vi "N664_Init.vi"() -> (1 "Status":bool, 2 "Positions":dbl[](array[numeric]), 3 "VISA Refnum out":refnum<visa-resource-name>)   [LabVIEW 2014]
uses:
  <vilib>/Instr/_visa.llb/VISA Configure Serial Port (Instr).vi
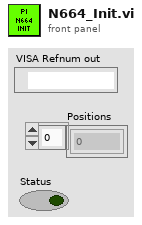
[diagram p1: front panel]
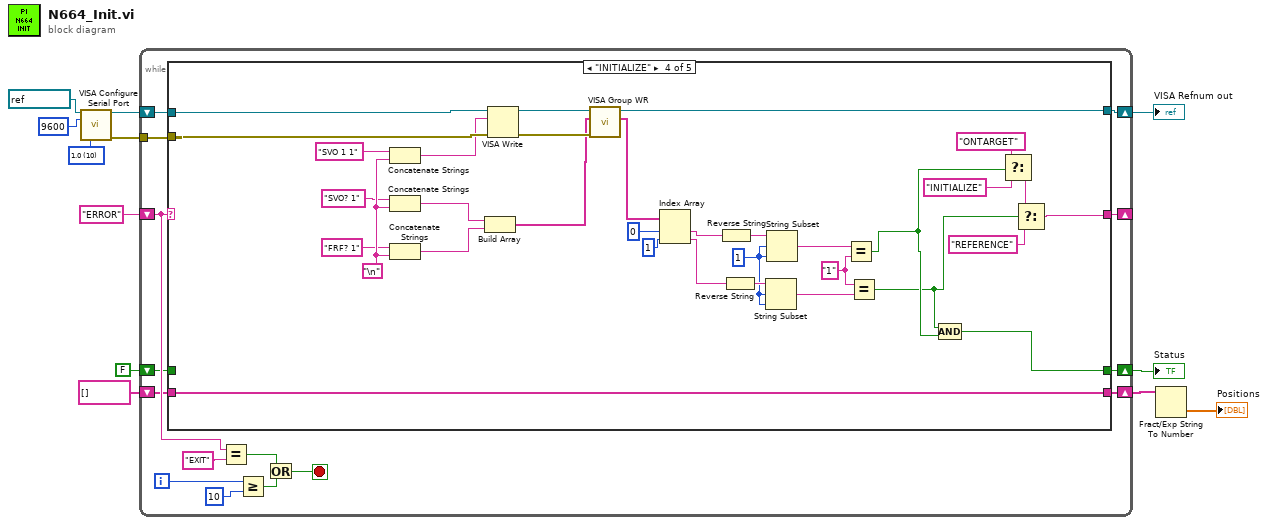
[diagram p0: block diagram]
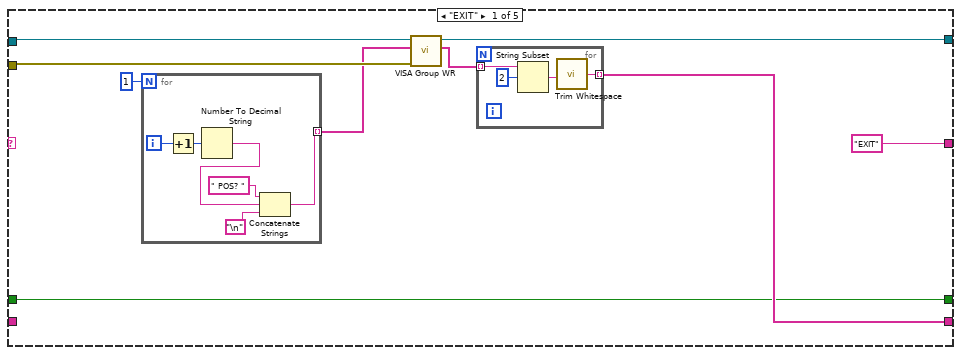
[diagram p2: hidden frame]
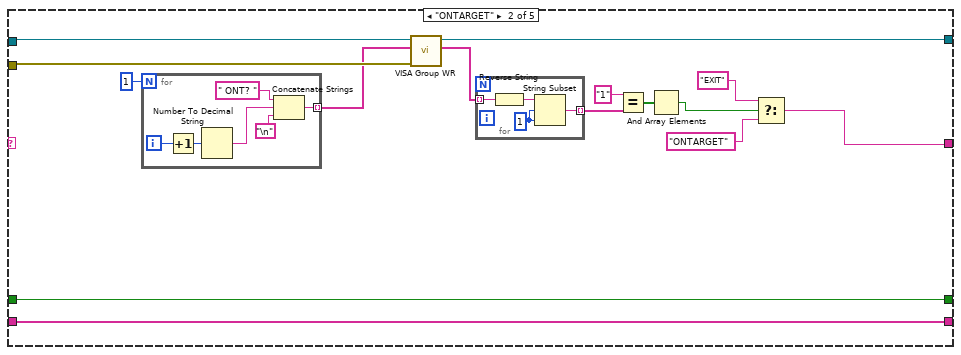
[diagram p3: hidden frame]
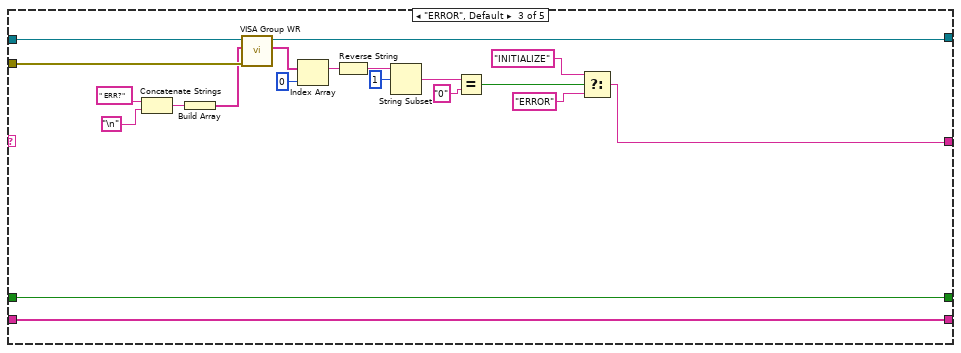
[diagram p4: hidden frame]
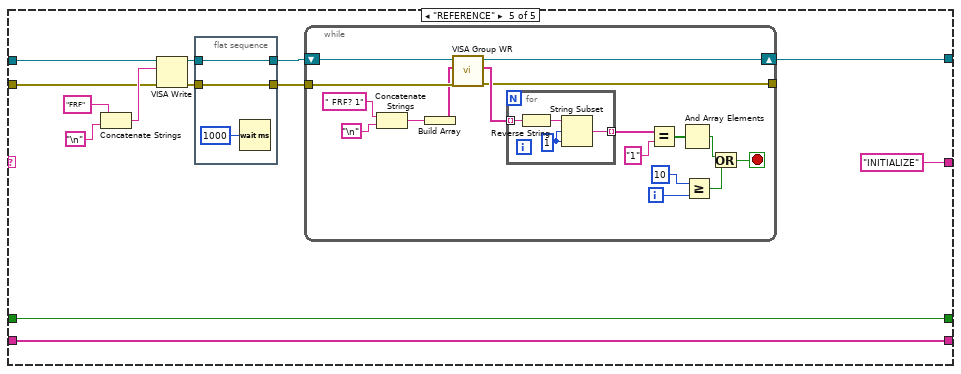
[diagram p5: hidden frame]
diagram:
  w8 = u16 10 items=["1.0"=10, "1.5"=15, "2.0"=20] ("stop bits (10: 1 bit)")
  n1 = call-poly "VISA Configure Serial Port"("VISA resource name"=refnum<visa-resource-name> "COM4", "baud rate (9600)"=u32 9600, "stop bits (10: 1 bit)"=w8) -> ("VISA resource name out"=w12:refnum<visa-resource-name>, "error out"=w9:errorcluster)  [unwired: 11 in]
  n2 = while {
    tunnel: w9 -> [w26]
    shift-right: [w25] -> _
    shift-left: "ERROR" -> [w23]
    shift-right: [w15] -> w5
    shift-left: w12 -> [w27]
    shift-right: [w16] -> w2
    shift-left: string[] [] -> [w14]
    shift-right: [w19] -> w11
    shift-left: FALSE -> [w13]
    i -> [w17]
    stop <- w21 stop-if-true
    n3 = case shown="\"INITIALIZE\"" w23 {
      tunnel: w27 -> [w35 w61 w89 w122 w134]
      tunnel: w26 -> [w34 w60 w88 w121 w133]
      tunnel: [w28 w48 w73 w103 w130] -> w19
      tunnel: ["EXIT" w49 w74 w109 "INITIALIZE"] -> w25
      tunnel: [w30 w47 w72 w101 w129] -> w16
      tunnel: [w29 w57 w79 w102 w131] -> w15
      tunnel: w14 -> [_ w47 w72 w101 w129]
      tunnel: w13 -> [w28 w48 w73 _ w130]
      frame "EXIT" {
        n4 = for {
          N: 1 -> [_]
          tunnel: [w46] -> w32 mode=indexing
          i -> [w43]
          n5 = Increment(x=w43) -> (x+1=w44:i32)
          n6 = Number To Decimal String(number=w44) -> (decimal integer string=w41:string)  [unwired: 1 in]
          n7 = Concatenate Strings(" POS? " ("string"), w41, "\n") -> (w46:string)
        }
        n8 = call "VISA Group WR.vi"("error in (no error)"=w34, "Array in"=w32, "VISA Refnum in"=w35) -> ("Array out"=w31:string[], "VISA Refnum out"=w29:refnum<visa-resource-name>)  [unwired: 6 in, 1 out]
        n9 = for {
          tunnel: w31 -> [w40] mode=indexing
          tunnel: [w37] -> w30 mode=indexing
          n10 = String Subset(string=w40, offset (0)=2) -> (substring=w38:string)  [unwired: 1 in]
          n11 = call <vilib>:"Trim Whitespace.vi"("string"=w38) -> ("trimmed string"=w37:string)  [unwired: 1 in]
        }
      }
      frame "ONTARGET" {
        n12 = for {
          N: 1 -> [_]
          tunnel: [w71] -> w58 mode=indexing
          i -> [w68]
          n13 = Increment(x=w68) -> (x+1=w69:i32)
          n14 = Number To Decimal String(number=w69) -> (decimal integer string=w66:string)  [unwired: 1 in]
          n15 = Concatenate Strings(" ONT? " ("string"), w66, "\n") -> (w71:string)
        }
        n16 = call "VISA Group WR.vi"("error in (no error)"=w60, "Array in"=w58, "VISA Refnum in"=w61) -> ("Array out"=w54:string[], "VISA Refnum out"=w57:refnum<visa-resource-name>)  [unwired: 6 in, 1 out]
        n17 = for {
          tunnel: [w62] -> _ mode=indexing
          tunnel: [w63] -> w55 mode=indexing
          tunnel: w54 -> [w62] mode=indexing
          w64 = 1 ("length (rest)")
          n18 = Reverse String(1:w62) -> (0:w65:string)
          n19 = String Subset(string=w65, offset (0)=w64, length (rest)=w64) -> (substring=w63:string)
        }
        n20 = Equal?(x="1", y=w55) -> (x = y?=w56:bool[])
        n21 = And Array Elements(Boolean array=w56) -> (logical AND=w52:bool)
        n22 = Select(t="EXIT", s=w52, f="ONTARGET") -> (s? t:f=w49:string)
      }
      frame "ERROR", Default {
        n23 = Concatenate Strings(" ERR?" ("string"), "\n") -> (w87:string)
        n24 = Build Array(w87) -> (w86:string[])
        n25 = call "VISA Group WR.vi"("error in (no error)"=w88, "Array in"=w86, "VISA Refnum in"=w89) -> ("Array out"=w82:string[], "VISA Refnum out"=w79:refnum<visa-resource-name>)  [unwired: 6 in, 1 out]
        n26 = Index Array(array=w82, index=0) -> (element=w81:string)
        n27 = Reverse String(1:w81) -> (0:w83:string)
        n28 = String Subset(string=w83, offset (0)=1) -> (substring=w85:string)  [unwired: 1 in]
        n29 = Equal?(x=w85, y="0") -> (x = y?=w77:bool)
        n30 = Select(t="INITIALIZE", s=w77, f="ERROR") -> (s? t:f=w74:string)
      }
      frame "INITIALIZE" {
        w94 = 1 ("length (rest)")
        w100 = "\n"
        w107 = "1"
        n31 = Concatenate Strings("SVO 1 1" ("string"), w100) -> (w120:string)
        n32 = Concatenate Strings("SVO? 1" ("string"), w100) -> (w119:string)
        n33 = Concatenate Strings("FRF? 1" ("string"), w100) -> (w118:string)
        n34 = Build Array(w119, w118) -> (w117:string[])
        n35 = VISA Write(VISA resource name=w122, write buffer=w120, error in (no error)=w121) -> (VISA resource name out=w123:refnum<visa-resource-name>, error out=w124:errorcluster)  [unwired: 1 out]
        n36 = call "VISA Group WR.vi"("error in (no error)"=w124, "Array in"=w117, "VISA Refnum in"=w123) -> ("Array out"=w110:string[], "VISA Refnum out"=w102:refnum<visa-resource-name>)  [unwired: 6 in, 1 out]
        n37 = Index Array(array=w110, index #1=0 ("index (row)"), index #2=1 ("index (row)")) -> (element #1=w113:string, element #2=w114:string)
        n38 = Reverse String(1:w113) -> (0:w96:string)
        n39 = Reverse String(1:w114) -> (0:w95:string)
        n40 = String Subset(string=w95, offset (0)=w94, length (rest)=w94) -> (substring=w108:string)
        n41 = String Subset(string=w96, offset (0)=w94, length (rest)=w94) -> (substring=w115:string)
        n42 = Equal?(x=w115, y=w107) -> (x = y?=w93:bool)
        n43 = Equal?(x=w107, y=w108) -> (x = y?=w92:bool)
        n44 = Compound Arithmetic op=AND(w92, w93) -> (w103:bool)
        n45 = Select(t="ONTARGET", s=w93, f="INITIALIZE") -> (s? t:f=w104:string)
        n46 = Select(t=w104, s=w92, f="REFERENCE") -> (s? t:f=w109:string)
      }
      frame "REFERENCE" {
        n47 = Concatenate Strings("FRF" ("string"), "\n") -> (w135:string)
        n48 = VISA Write(VISA resource name=w134, write buffer=w135, error in (no error)=w133) -> (VISA resource name out=w127:refnum<visa-resource-name>, error out=w125:errorcluster)  [unwired: 1 out]
        n49 = flat-sequence {
          tunnel: [w140] -> w128
          tunnel: w127 -> [w140]
          tunnel: [w138] -> w126
          tunnel: w125 -> [w138]
          frame #0 {
            n50 = Wait (ms)(milliseconds to wait=u32 1000) -> ()  [unwired: 1 out]
          }
        }
        n51 = while {
          tunnel: w126 -> [w149]
          tunnel: [w148] -> _
          shift-right: [w156] -> w131
          shift-left: w128 -> [w157]
          i -> [w147]
          stop <- w145 stop-if-true
          n52 = Concatenate Strings(" FRF? 1" ("string"), "\n") -> (w155:string)
          n53 = Build Array(w155) -> (w142:string[])
          n54 = call "VISA Group WR.vi"("error in (no error)"=w149, "Array in"=w142, "VISA Refnum in"=w157) -> ("error out"=w148:errorcluster, "Array out"=w154:string[], "VISA Refnum out"=w156:refnum<visa-resource-name>)  [unwired: 6 in]
          n55 = for {
            tunnel: w154 -> [w159] mode=indexing
            tunnel: [w158] -> w151 mode=indexing
            w161 = 1 ("length (rest)")
            n56 = Reverse String(1:w159) -> (0:w160:string)
            n57 = String Subset(string=w160, offset (0)=w161, length (rest)=w161) -> (substring=w158:string)
          }
          n58 = Equal?(x=w151, y="1") -> (x = y?=w152:bool[])
          n59 = And Array Elements(Boolean array=w152) -> (logical AND=w150:bool)
          n60 = Greater Or Equal?(x=10, y=w147) -> (x >= y?=w144:bool)
          n61 = Or(x=w150, y=w144) -> (x .or. y?=w145:bool)
        }
      }
    }
    n62 = Equal?(x=w23, y="EXIT") -> (x = y?=w22:bool)
    n63 = Greater Or Equal?(x=w17, y=10 ("x")) -> (x >= y?=w20:bool)
    n64 = Or(x=w22, y=w20) -> (x .or. y?=w21:bool)
  }
  "VISA Refnum out" <- w5
  "Status" <- w11
  n65 = Fract/Exp String To Number(string=w2) -> (number=→"Positions":dbl[])  [unwired: 3 in, 1 out]
